vi "scada.vi"() -> ()   [LabVIEW 2014]
panel:
  out "Waveform Chart":dynamicdata(graph)
  in  "STOP":bool
  out "PV":dbl
  in  "Ref":dbl=8.0
  in  "Ki":dbl=2.0
  in  "Kp":dbl=4.0
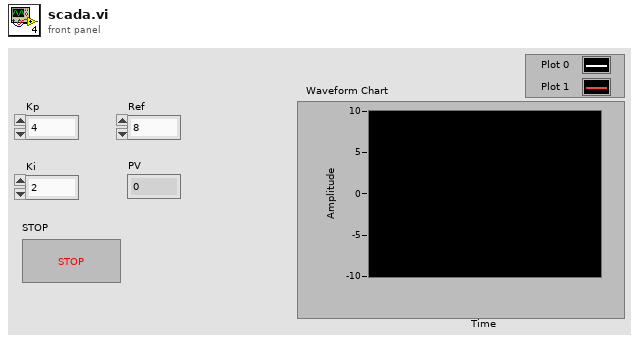
[diagram p1: front panel]
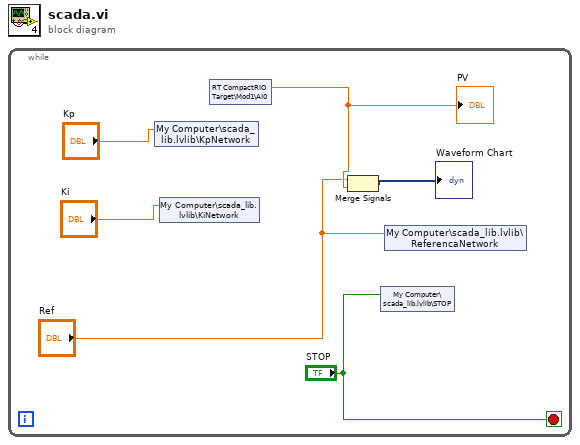
[diagram p0: block diagram]
diagram:
  n1 = while {
    stop <- "STOP" stop-if-true
    n2 = shared-variable "My Computer\\scada_lib.lvlib\\KpNetwork"("Kp") -> ()  [unwired: 1 in, 1 out]
    n3 = shared-variable "My Computer\\scada_lib.lvlib\\KiNetwork"("Ki") -> ()  [unwired: 1 in, 1 out]
    n4 = shared-variable "RT CompactRIO Target\\Mod1\\AI0"() -> (w3:dbl)  [unwired: 1 in, 1 out]
    "PV" <- w3
    n5 = Merge Signals("Ref", w3) -> (→"Waveform Chart":dynamicdata)
    n6 = shared-variable "My Computer\\scada_lib.lvlib\\STOP"("STOP") -> ()  [unwired: 1 in, 1 out]
    n7 = shared-variable "My Computer\\scada_lib.lvlib\\ReferencaNetwork"("Ref") -> ()  [unwired: 1 in, 1 out]
  }
